vi "Release.vi"(8 "error in (no error)":errorcluster, 11 "UI_ProgressBar in":refnum<class "UI_ProgressDlg.lvclass">) -> (0 "error out":errorcluster, 3 "UI_ProgressBar out":refnum<class "UI_ProgressDlg.lvclass">)   [LabVIEW 2014, in "UI_ProgressDlg.lvlib" / "UI_ProgressDlg.lvclass"]
uses:
  UI_ProgressDlg.lvclass
  UI_ProgressDlg.lvclass/UI_ProgressDlg.ctl
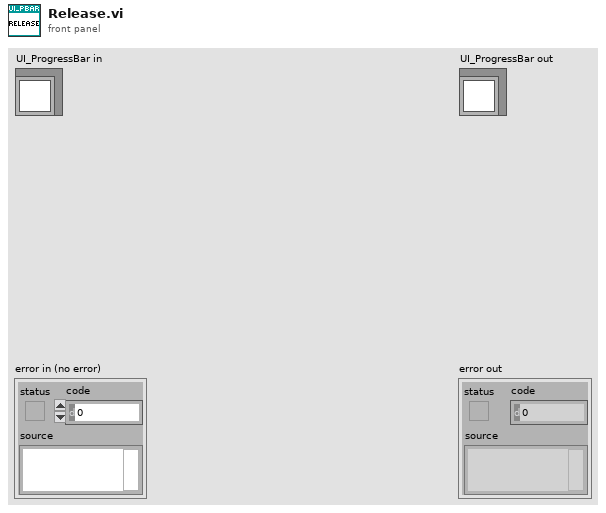
[diagram p1: front panel]
types:
  T1 = enum32{"Invalid", "Standard", "Closed", "Hidden", "Minimized", "Maximized"}
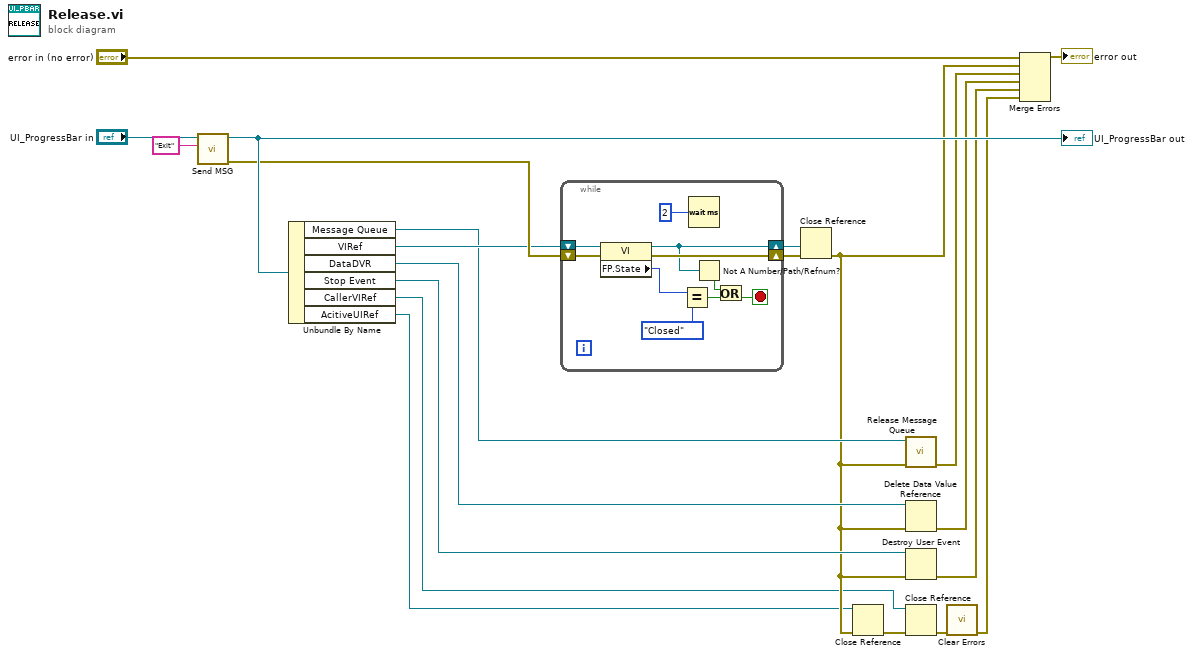
[diagram p0: block diagram]
diagram:
  n1 = call "Send MSG.vi"("msg"="Exit", "UI_ProgressBar in"="UI_ProgressBar in") -> ("error out"=w18:errorcluster, "UI_ProgressBar out"=w20:refnum<class "UI_ProgressDlg.lvclass">)  [unwired: 8 in]
  "UI_ProgressBar out" <- w20
  n2 = Unbundle By Name(w20) -> ("Message Queue"=w12:refnum<queue>, "VIRef"=w15:refnum<vi>, "DataDVR"=w10:refnum<data-value>, "Stop Event"=w8:refnum<user-event>, "CallerVIRef"=w2:refnum<vi>, "AcitiveUIRef"=w3:refnum<vi>)
  n3 = while {
    shift-right: [w22] -> w14
    shift-left: w15 -> [w31]
    shift-right: [w29] -> w13
    shift-left: w18 -> [w30]
    stop <- w24 stop-if-true
    n4 = property class="VI"(reference=w31, error in=w30) -> (reference out=w22:refnum<vi>, error out=w29:errorcluster, "FP.State"=w28:T1)
    n5 = Equal?(x=w28, y=T1."Closed") -> (x = y?=w27:bool)
    n6 = Wait (ms)(milliseconds to wait=u32 2) -> ()  [unwired: 1 out]
    n7 = Not A Number/Path/Refnum?(number/path/refnum=w22) -> (NaN/Path/Refnum?=w23:bool)
    n8 = Or(x=w23, y=w27) -> (x .or. y?=w24:bool)
  }
  n9 = Close Reference(reference=w14, error in (no error)=w13) -> (error out=w6:errorcluster)
  n10 = Close Reference(reference=w3, error in (no error)=w6) -> (error out=w5:errorcluster)
  n11 = call "Release Message Queue.vi"("error in (no error)"=w6, "Message Queue"=w12) -> ("error out"=w11:errorcluster)  [unwired: 9 in]
  n12 = Delete Data Value Reference(data value reference=w10, error in=w6) -> (error out=w9:errorcluster)  [unwired: 1 out]
  n13 = Destroy User Event(user event=w8, error in=w6) -> (error out=w7:errorcluster)
  n14 = Close Reference(reference=w2, error in (no error)=w5) -> (error out=w4:errorcluster)
  n15 = call <vilib>:"Clear Errors.vi"("error in (no error)"=w4) -> ("error out"=w1:errorcluster)  [unwired: 5 in, 1 out]
  n16 = Merge Errors("error in (no error)", w6, w11, w9, w7, w1) -> (→"error out":errorcluster)
